vi "sort name by time.vi"(6 "time format":string="%<%Y-%m-%d-%%Hh%Mm%Ss%3u>T", 8 "error in (no error)":errorcluster, 10 "filenames":string[](array[string])) -> (0 "error out":errorcluster, 2 "sorted filename":string[](array[string]))   [LabVIEW 2019]
doc: "scan a 1D string element by element to scan a time and date patern and short the array by it.\n\ntime format: the time format scan like %<%Y-%m-%d-%%Hh%Mm%Ss%3u>T"
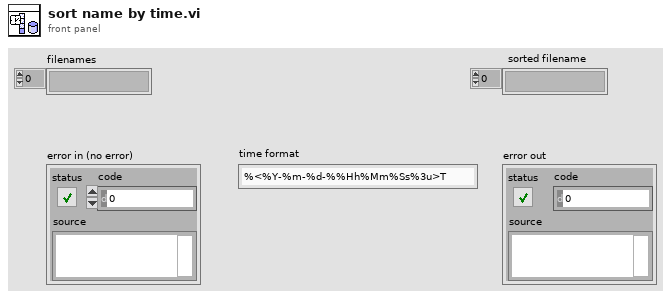
[diagram p1: front panel]
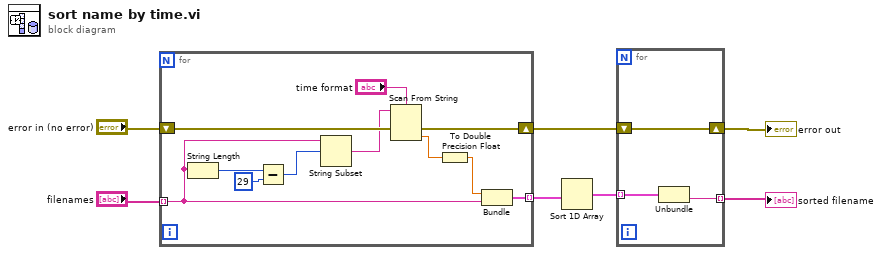
[diagram p0: block diagram]
diagram:
  n1 = for {
    shift-right: [w18] -> w1
    shift-left: "error in (no error)" -> [w17]
    tunnel: "filenames" -> [w11] mode=indexing
    tunnel: [w10] -> w6 mode=indexing
    n2 = String Length(string=w11) -> (length=w16:i32)
    n3 = Subtract(x=w16, y=29) -> (x-y=w14:i32)
    n4 = String Subset(string=w11, offset (0)=w14) -> (substring=w13:string)  [unwired: 1 in]
    n5 = Scan From String(format string="time format", input string=w13, error in=w17) -> (error out=w18:errorcluster, output 1=w9:dbl)  [unwired: 2 in, 2 out]
    n6 = To Double Precision Float(number=w9) -> (double precision float=w12:dbl)
    n7 = Bundle(w12, w11) -> (w10:cluster{dbl, string})  [unwired: 1 in]
  }
  n8 = Sort 1D Array(array=w6) -> (sorted array=w7:cluster{dbl, string}[])
  n9 = for {
    tunnel: w7 -> [w21] mode=indexing
    tunnel: [w20] -> w3 mode=indexing
    shift-right: [w19] -> w2
    shift-left: w1 -> [w19]
    n10 = Unbundle(w21) -> (w20:string)  [unwired: 1 out]
  }
  "error out" <- w2
  "sorted filename" <- w3
